vi "Character_Create.vi"(7 "Character":string, 8 "error in (no error)":errorcluster, 9 "Color":u32, 10 "Font":T1, 11 "reference in":refnum<class "Character.lvclass">) -> (0 "error out":errorcluster, 3 "reference out":refnum<class "Character.lvclass">)   [LabVIEW 2012, in "Character.lvclass"]
uses:
  Character.lvclass
  Glyph_class/Glyph.lvclass
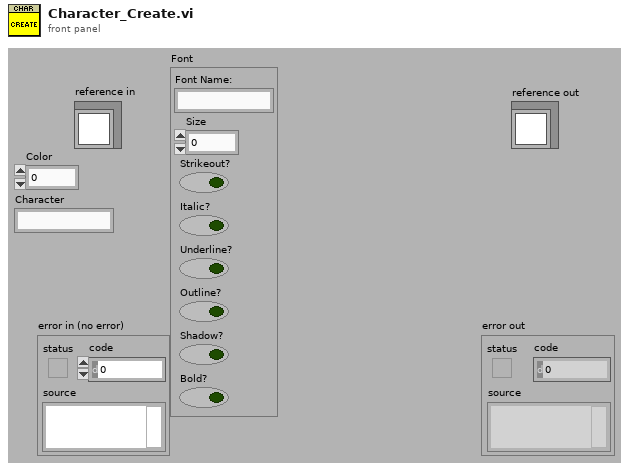
[diagram p1: front panel]
types:
  T1 = cluster{"Font Name:":string, "Size":i16, "Strikeout?":bool, "Italic?":bool, "Underline?":bool, "Outline?":bool, "Shadow?":bool, "Bold?":bool}
  T2 = typedef "Character.lvclass/ObjectAttributes.ctl" = cluster{"Font":cluster{"Font Name:":string, "Size":i16, "Strikeout?":bool, "Italic?":bool, "Underline?":bool, "Outline?":bool, "Shadow?":bool, "Bold?":bool}, "Color":u32, "Character":string}
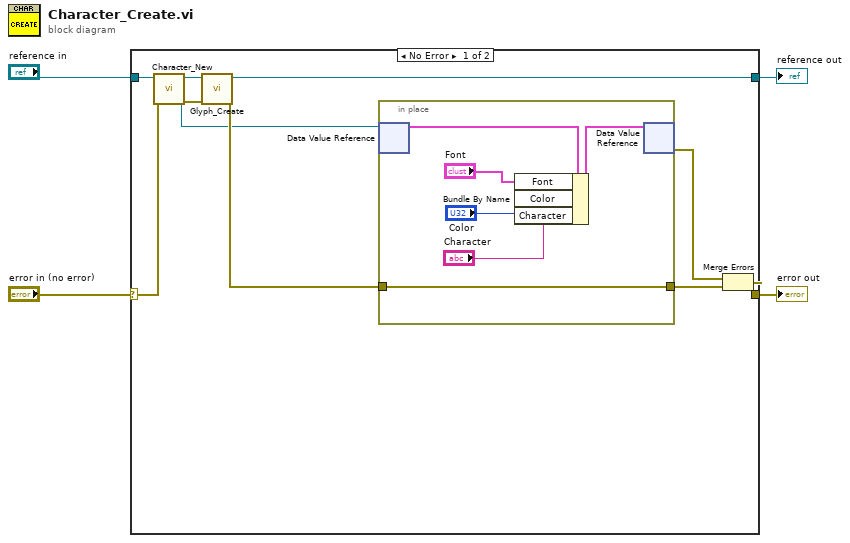
[diagram p0: block diagram]
diagram:
  n1 = case shown="No Error" "error in (no error)" {
    selector: "error in (no error)" -> [w8 w22]
    tunnel: [w12 w22] -> w3
    tunnel: "reference in" -> [w9 w21]
    tunnel: [w14 w21] -> w1
    frame No Error {
      n2 = call "Character_New.vi"("error in (no error)"=w8, "reference in"=w9) -> ("error out"=w6:errorcluster, "DVRRefOut"=w5:refnum<data-value>, "reference out"=w7:refnum<class "Character.lvclass">)  [unwired: 6 in, 1 out]
      n3 = call "Glyph_Create.vi"("error in (no error)"=w6, "reference in"=w7) -> ("error out"=w11:errorcluster, "reference out"=w14:refnum<class "Character.lvclass">)  [unwired: 8 in]
      n4 = in-place {
        in-place-border: w11 -> [w18]
        in-place-border: [w18] -> w10
        n5 = in-place-dvr #1(w5) -> (w19:T2)  [unwired: 1 out]
        n6 = Bundle By Name(cluster=w19, "Font"="Font", "Color"="Color", "Character"="Character") -> (w20:T2)
        n7 = in-place-dvr #1(w20) -> (w13:errorcluster)  [unwired: 1 out]
      }
      n8 = Merge Errors(w13, w10) -> (w12:errorcluster)
    }
    frame Error {
    }
  }
  "error out" <- w3
  "reference out" <- w1
